vi "Save Config File.vi"(8 "error in (no error)":errorcluster, 10 "file path":path, 11 "queue in":refnum<queue>) -> (0 "error out":errorcluster, 2 "file path out":path, 3 "queue out":refnum<queue>)   [LabVIEW 2017, in "NI_LVConfig.lvlib"]
uses:
  NI_LVConfig.lvlib
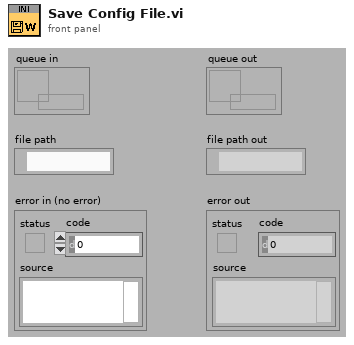
[diagram p1: front panel]
types:
  T1 = enum16{"open", "replace", "create", "open or create", "replace or create", "replace or create with confirmation"}
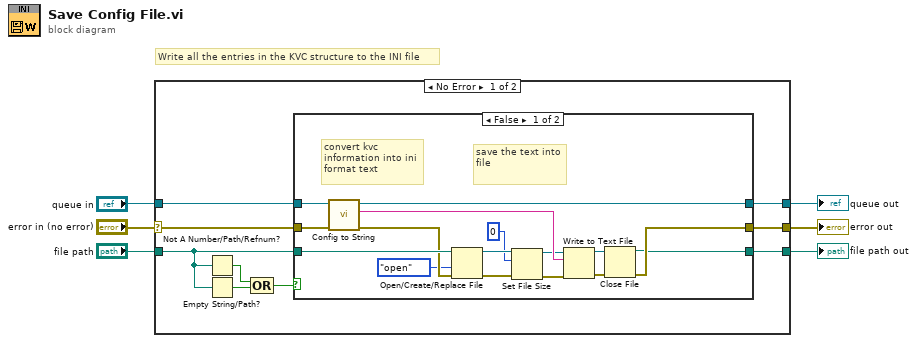
[diagram p0: block diagram]
diagram:
  # "Write all the entries in the KVC structure to the INI file"
  n1 = case shown="No Error" "error in (no error)" {
    selector: "error in (no error)" -> [w8 w37]
    tunnel: [w15 w37] -> w5
    tunnel: [w14 w36] -> w3
    tunnel: "queue in" -> [w9 w36]
    tunnel: "file path" -> [w10 w35]
    tunnel: [w7 w35] -> w1
    frame No Error {
      n2 = Not A Number/Path/Refnum?(number/path/refnum=w10) -> (NaN/Path/Refnum?=w13:bool)
      n3 = Empty String/Path?(string/path=w10) -> (empty?=w12:bool)
      n4 = Compound Arithmetic op=OR(w13, w12) -> (w11:bool)
      n5 = case shown="False" w11 {
        tunnel: [w29 w34] -> w15
        tunnel: w8 -> [w25 w34]
        tunnel: w10 -> [w26 w32]
        tunnel: w9 -> [w27 w33]
        tunnel: [w22 w33] -> w14
        tunnel: [w21 w32] -> w7
        frame False {
          # "save the text into file"
          # "convert kvc information into ini format text"
          n6 = call "Config to String.vi"("error in (no error)"=w25, "queue in"=w27) -> ("error out"=w24:errorcluster, "String"=w28:string, "queue out"=w22:refnum<queue>)  [unwired: 7 out]
          n7 = Open/Create/Replace File(file path (use dialog)=w26, error in=w24, operation (0:open)=T1."open") -> (refnum out=w18:refnum<file>, error out=w20:errorcluster)  [unwired: 4 out]
          n8 = Set File Size(4:w20, 6:i64 0 ("size (in bytes)"), 7:w18) -> (0:w19:errorcluster, 3:w17:refnum<file>)
          n9 = Write to Text File(file (use dialog)=w17, text=w28, error in=w19) -> (refnum out=w31:refnum<file>, error out=w30:errorcluster)  [unwired: 2 out]
          n10 = Close File(refnum=w31, error in=w30) -> (path=w21:path, error out=w29:errorcluster)
        }
        frame True {
        }
      }
    }
    frame Error {
    }
  }
  "error out" <- w5
  "queue out" <- w3
  "file path out" <- w1
